vi "Scan Engine EtherCAT Generic Slave.vi"(8 "error in (no error)":errorcluster, 11 "Node Ptr":T1 format="%.0x") -> (0 "error out":errorcluster)   [LabVIEW 2020, in "SEECD System Explorer.lvlib"]
uses:
  SEECD System Explorer.lvlib
  <vilib>/NI VeriStand/Custom Device API/Custom Device API.lvlib
  NationalInstruments.VeriStand.SystemDefinitionAPI
  Shared/Globals/Property Strings.vi
  Shared/SEECD Shared.lvlib
  <vilib>/NI VeriStand/Custom Device API/Set Item Property (Boolean).vi
  <vilib>/NI VeriStand/Custom Device API/Custom Device Item Ref.ctl
panel:
  in  "Enable Distributed Clock":bool caption="Enable distributed clock"
  out "ToString":string
  in  "Export to XML":bool
  in  "Prepend":bool caption="Prepend slave position to name"
  in  "SHDocVw.IWebBrowser2":refnum<k7>(container)
  in  "Slave Position":u16
  in  "Header":cluster{"Section Name":string}={"Section Name"="EtherCAT Slave"}
  in  "Name":string
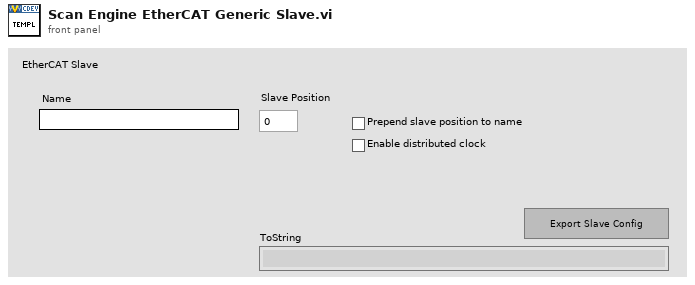
[diagram p1: front panel]
types:
  T1 = typedef "Custom Device API.lvlib/Custom Device Item Ref.ctl" = u64
  T2 = typedef "Custom Device API.lvlib/Custom Device Commands.ctl" = enum16{"Default", "Item renamed", "Shutdown", "Dynamic button pressed"}
  T3 = typedef "Custom Device API.lvlib/Custom Device Pointer.ctl" = refnum<k24>
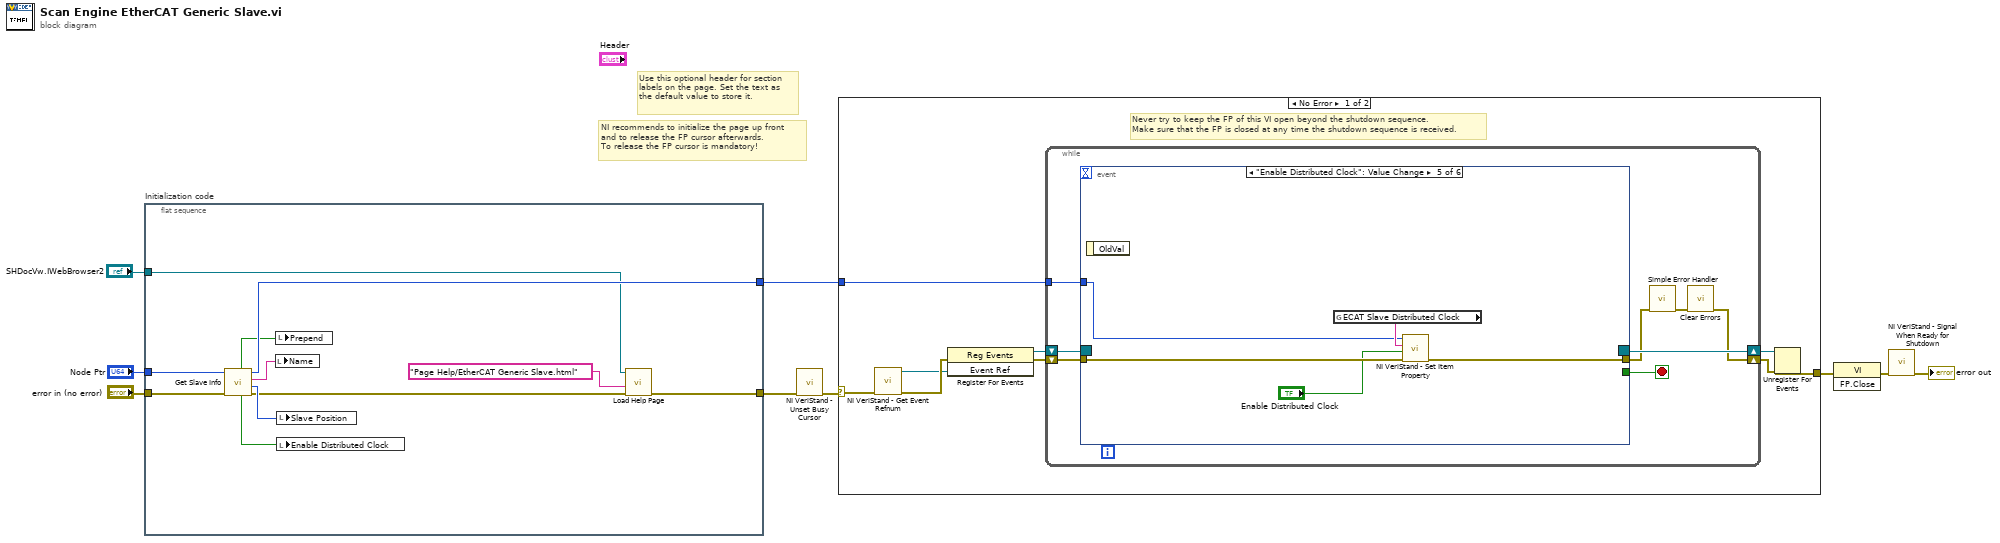
[diagram p0: block diagram]
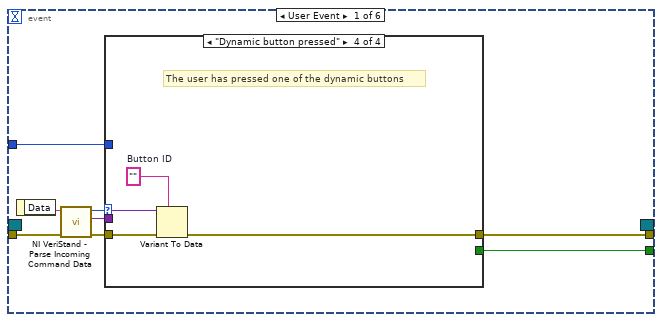
[diagram p2: hidden frame]
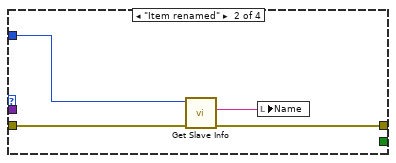
[diagram p4: hidden frame]
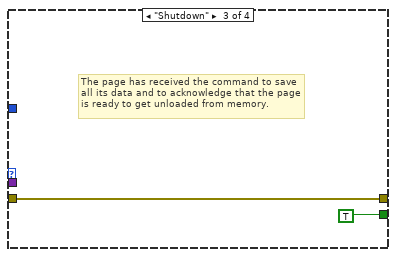
[diagram p5: hidden frame]
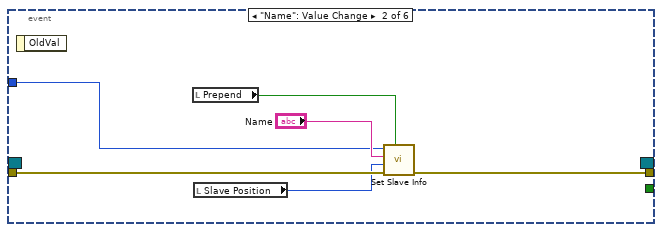
[diagram p6: hidden frame]
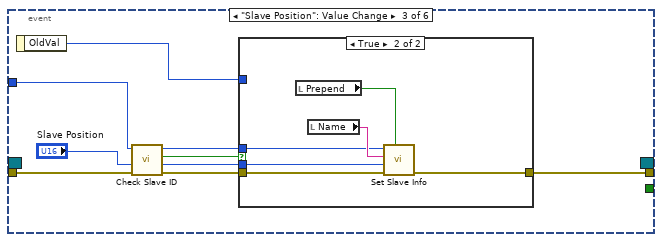
[diagram p7: hidden frame]
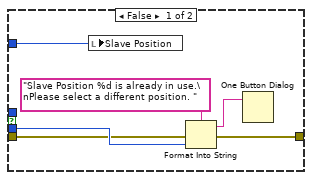
[diagram p8: hidden frame]
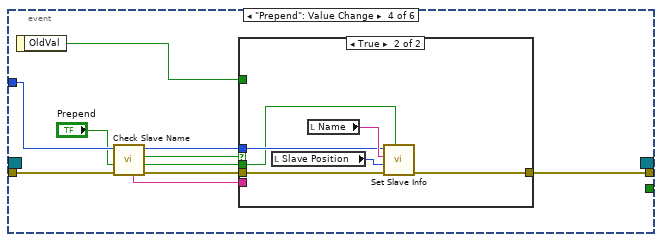
[diagram p9: hidden frame]
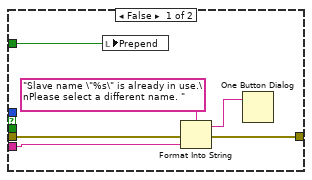
[diagram p10: hidden frame]
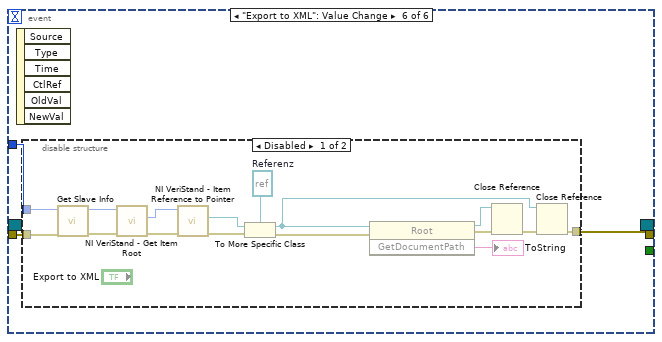
[diagram p11: hidden frame]
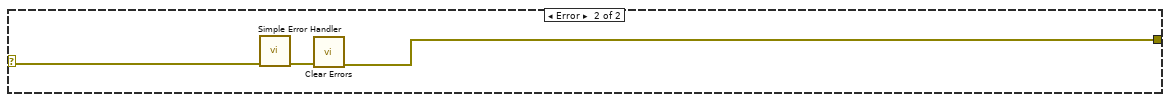
[diagram p13: hidden frame]
diagram:
  # "Use this optional header for section labels on the page. Set the text as the default value to store it."
  # "NI recommends to initialize the page up front\nand to release the FP cursor afterwards.\nTo release the FP cursor is mandatory!"
  n1 = flat-sequence "Initialization code" {
    tunnel: "error in (no error)" -> [w16]
    tunnel: "Node Ptr" -> [w17]
    tunnel: [w18] -> w3
    tunnel: "SHDocVw.IWebBrowser2" -> [w11]
    tunnel: [w12] -> w1
    frame #0 {
      n2 = call "Get Slave Info.vi"("error in (no error)"=w16, "Item Ref in"=w17) -> ("error out"=w13:errorcluster, "Slave #"=w19:u16, "Slave Name"=w20:string, "Item Ref out"=w18:T1, "Distributed Clock"=w10:bool, "Prepend"=w15:bool)  [unwired: 4 in]
      n3 = local write "Name"(w20) -> ()
      n4 = local write "Prepend"(w15) -> ()
      n5 = local write "Slave Position"(w19) -> ()
      n6 = local write "Enable Distributed Clock"(w10) -> ()
      n7 = call "Load Help Page.vi"("error in (no error)"=w13, "HTML File to Load"="Page Help/EtherCAT Generic Slave.html" ("name or relative path"), "Browser"=w11) -> ("error out"=w12:errorcluster)  [unwired: 8 in]
    }
  }
  n8 = call <vilib>:"NI VeriStand - Unset Busy Cursor.vi"("error in (no error)"=w1) -> ("error out"=w5:errorcluster)  [unwired: 10 out]
  n9 = case shown="No Error" w5 {
    selector: w5 -> [w21 w132]
    tunnel: [w26 w130] -> w9
    tunnel: w3 -> [w22 _]
    frame No Error {
      # "Never try to keep the FP of this VI open beyond the shutdown sequence.\nMake sure that the FP is closed at any time the shutdown sequence is received."
      n10 = call <vilib>:"NI VeriStand - Get Event Refnum.vi"("error in (no error)"=w21) -> ("error out"=w29:errorcluster, "Event Ref"=w25:refnum<user-event>)  [unwired: 9 out]
      n11 = register-events(error in=w29, w25) -> (reference out=w23:refnum<event-registration>, error out=w24:errorcluster)  [unwired: 1 in]
      n12 = while {
        tunnel: w22 -> [w33]
        shift-right: [w30] -> w27
        shift-left: w24 -> [w36]
        shift-right: [w37] -> w28
        shift-left: w23 -> [w35]
        stop <- w34 stop-if-true
        n13 = event shown="[4] \"Enable Distributed Clock\": Value Change" {
          selector: w35 -> [_ _ _ _ _ _]
          dyn-events: [_ _ _ _ _ _] -> w37
          timeout: _ -> [_ _ _ _ _ _]
          tunnel: w36 -> [w45 w60 w65 w91 w109 w113]
          tunnel: [w41 _ _ _ _ _] -> w34
          tunnel: [w40 w61 w63 w92 w108 w111] -> w32
          tunnel: w33 -> [w39 w59 w67 w90 w107 w112]
          event User Event {
            n14 = event-data() -> ("Data"=w44:string)  [unwired: 1 out]
            n15 = call <vilib>:"NI VeriStand - Parse Incoming Command Data.vi"("error in (no error)"=w45, "Incoming data"=w44) -> ("error out"=w43:errorcluster, "Outgoing data"=w38:variant, "Action"=w42:T2)  [unwired: 7 out]
            n16 = case shown="\"Dynamic button pressed\"" w42 {
              tunnel: w43 -> [w46 w50 w51 w56]
              tunnel: [_ _ TRUE _] -> w41
              tunnel: [w46 w49 w51 w53] -> w40
              tunnel: w39 -> [_ w47 _ _]
              tunnel: w38 -> [_ _ _ w55]
              frame "Default", Default {
              }
              frame "Item renamed" {
                n17 = call "Get Slave Info.vi"("error in (no error)"=w50, "Item Ref in"=w47) -> ("error out"=w49:errorcluster, "Slave Name"=w48:string)  [unwired: 4 in, 4 out]
                n18 = local write "Name"(w48) -> ()
              }
              frame "Shutdown" {
                # "The page has received the command to save all its data and to acknowledge that the page is ready to get unloaded from memory."
              }
              frame "Dynamic button pressed" {
                w54 = ""  # Button ID
                # "The user has pressed one of the dynamic buttons"
                n19 = Variant To Data(error in=w56, type=w54, Variant=w55) -> (error out=w53:errorcluster)  [unwired: 1 out]
              }
            }
          }
          event "Name": Value Change {
            n20 = event-data() -> ()  [unwired: 2 out]
            n21 = local read "Prepend"() -> (w57:bool)
            n22 = local read "Slave Position"() -> (w58:u16)
            n23 = call "Set Slave Info.vi"("Prepend"=w57, "error in (no error)"=w60, "Slave #"=w58, "Slave Name"="Name", "Item Ref in"=w59) -> ("error out"=w61:errorcluster)  [unwired: 5 in, 1 out]
          }
          event "Slave Position": Value Change {
            n24 = event-data() -> ("OldVal"=w64:u16)  [unwired: 1 out]
            n25 = call "Check Slave ID.vi"("error in (no error)"=w65, "Slave ID in"="Slave Position", "Item Ref in"=w67) -> ("error out"=w71:errorcluster, "Slave ID out"=w69:u16, "Available?"=w70:bool, "Item Ref out"=w68:T1)  [unwired: 5 in]
            n26 = case shown="True" w70 {
              tunnel: [w73 w83] -> w63
              tunnel: w71 -> [w74 w82]
              tunnel: w68 -> [_ w79]
              tunnel: w69 -> [w76 w81]
              tunnel: w64 -> [w72 _]
              frame False {
                n27 = local write "Slave Position"(w72) -> ()
                n28 = Format Into String(format string="Slave Position %d is already in use.\nPlease select a different position. ", error in=w74, w76) -> (resulting string=w75:string, error out=w73:errorcluster)  [unwired: 1 in]
                n29 = One Button Dialog(message=w75) -> ()  [unwired: 1 in, 1 out]
              }
              frame True {
                n30 = local read "Prepend"() -> (w78:bool)
                n31 = local read "Name"() -> (w80:string)
                n32 = call "Set Slave Info.vi"("Prepend"=w78, "error in (no error)"=w82, "Slave #"=w81, "Slave Name"=w80, "Item Ref in"=w79) -> ("error out"=w83:errorcluster)  [unwired: 5 in, 1 out]
              }
            }
          }
          event "Prepend": Value Change {
            n33 = event-data() -> ("OldVal"=w93:bool)  [unwired: 1 out]
            n34 = call "Check Slave Name.vi"("error in (no error)"=w91, "Prepend in"="Prepend", "Item Ref in"=w90) -> ("error out"=w86:errorcluster, "Prepend out"=w85:bool, "Available?"=w87:bool, "Item Ref out"=w88:T1, "Slave Name"=w84:string)  [unwired: 4 in]
            n35 = case shown="True" w87 {
              tunnel: [w96 w105] -> w92
              tunnel: w86 -> [w97 w104]
              tunnel: w88 -> [_ w102]
              tunnel: w85 -> [_ w101]
              tunnel: w93 -> [w99 _]
              tunnel: w84 -> [w94 _]
              frame False {
                n36 = local write "Prepend"(w99) -> ()
                n37 = Format Into String(format string="Slave name \"%s\" is already in use.\nPlease select a different name. ", error in=w97, w94) -> (resulting string=w95:string, error out=w96:errorcluster)  [unwired: 1 in]
                n38 = One Button Dialog(message=w95) -> ()  [unwired: 1 in, 1 out]
              }
              frame True {
                n39 = local read "Slave Position"() -> (w100:u16)
                n40 = local read "Name"() -> (w103:string)
                n41 = call "Set Slave Info.vi"("Prepend"=w101, "error in (no error)"=w104, "Slave #"=w100, "Slave Name"=w103, "Item Ref in"=w102) -> ("error out"=w105:errorcluster)  [unwired: 5 in, 1 out]
              }
            }
          }
          event "Enable Distributed Clock": Value Change {
            n42 = event-data() -> ()  [unwired: 2 out]
            n43 = global read "Property Strings.vi" "ECAT Slave Distributed Clock"() -> (w110:string)
            n44 = call-poly <vilib>:"NI VeriStand - Set Item Property.vi"("error in (no error)"=w109, "Value"="Enable Distributed Clock", "Property Name"=w110, "Item Ref in"=w107) -> ("error out"=w108:errorcluster)  [unwired: 5 in, 2 out]
          }
          event "Export to XML": Value Change {
            n45 = event-data() -> ()  [unwired: 7 out]
            n46 = disable-structure shown="Disabled" {
              disable-tunnel: w113 -> [w129 _]
              disable-tunnel: w112 -> [w128 _]
              disable-tunnel: [w123 _] -> w111
              frame Disabled {
                w117 = refnum<k24> refnum  # Referenz
                n47 = call "Get Slave Info.vi"("error in (no error)"=w129, "Item Ref in"=w128) -> ("error out"=w127:errorcluster, "Item Ref out"=w119:T1)  [unwired: 4 in, 4 out]
                n48 = call <vilib>:"NI VeriStand - Get Item Root.vi"("error in (no error)"=w127, "Item Ref in"=w119) -> ("error out"=w120:errorcluster, "Root Ref out"=w116:T1)  [unwired: 6 in, 2 out]
                n49 = call <vilib>:"NI VeriStand - Item Reference to Pointer.vi"("error in (no error)"=w120, "Item Ref in"=w116) -> ("error out"=w122:errorcluster, "Node Pointer"=w115:T3)  [unwired: 6 in, 2 out]
                n50 = To More Specific Class(target class=w117, reference=w115, error in=w122) -> (specific class reference=w118:refnum<k24>, error out=w121:errorcluster)
                n51 = invoke class="Root" method="GetDocumentPath"(reference=w118, error in=w121) -> (reference out=w125:refnum<k24>, error out=w126:errorcluster, "GetDocumentPath"=→"ToString":string)  [unwired: 1 in]
                n52 = Close Reference(reference=w125, error in (no error)=w126) -> (error out=w124:errorcluster)
                n53 = Close Reference(reference=w118, error in (no error)=w124) -> (error out=w123:errorcluster)
              }
              frame Enabled {
              }
            }
          }
        }
        n54 = call <vilib>:"Simple Error Handler.vi"("error in (no error)"=w32) -> ("error out"=w31:errorcluster)  [unwired: 1 in, 7 out]
        n55 = call <vilib>:"Clear Errors.vi"("error in (no error)"=w31) -> ("error out"=w30:errorcluster)  [unwired: 1 in, 5 out]
      }
      n56 = Unregister For Events(event registration refnum=w28, error in=w27) -> (error out=w26:errorcluster)
    }
    frame Error {
      n57 = call <vilib>:"Simple Error Handler.vi"("error in (no error)"=w132) -> ("error out"=w131:errorcluster)  [unwired: 1 in, 7 out]
      n58 = call <vilib>:"Clear Errors.vi"("error in (no error)"=w131) -> ("error out"=w130:errorcluster)  [unwired: 1 in, 5 out]
    }
  }
  n59 = invoke class="VI" method="FP.Close"(error in=w9) -> (error out=w8:errorcluster)  [unwired: 2 in, 2 out]
  n60 = call <vilib>:"NI VeriStand - Signal When Ready for Shutdown.vi"("error in (no error)"=w8) -> ("error out"=→"error out":errorcluster)  [unwired: 10 out]
